vi "CreateMicron.vi"(8 "error in (no error)":errorcluster, 10 "New Microservice Name":string, 11 "Root Directory":path) -> (0 "error out":errorcluster, 3 "Project Path Out":path)   [LabVIEW 2019]
uses:
  <vilib>/SLL Toolkit/SLL Scripting/_Typedefs/Rename Item Cluster.ctl
  <vilib>/SLL Toolkit/SLL Scripting/SLL Scripting.lvlib
  <vilib>/SLL Toolkit/SLL Debug/SLL Debug.lvlib
panel:
  out "Micron Template Project Path":path
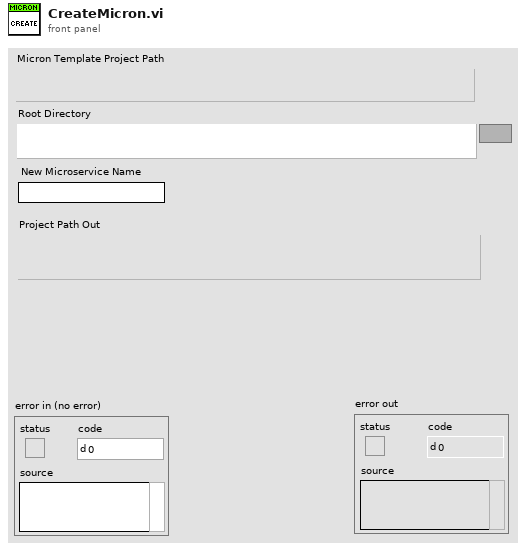
[diagram p1: front panel]
types:
  T1 = cluster{"Microservice Name":string, "Root Directory":path}
  T2 = typedef "SLL Scripting.lvlib/Rename Item Cluster.ctl" = cluster{"Existing":string, "Rename As":string}
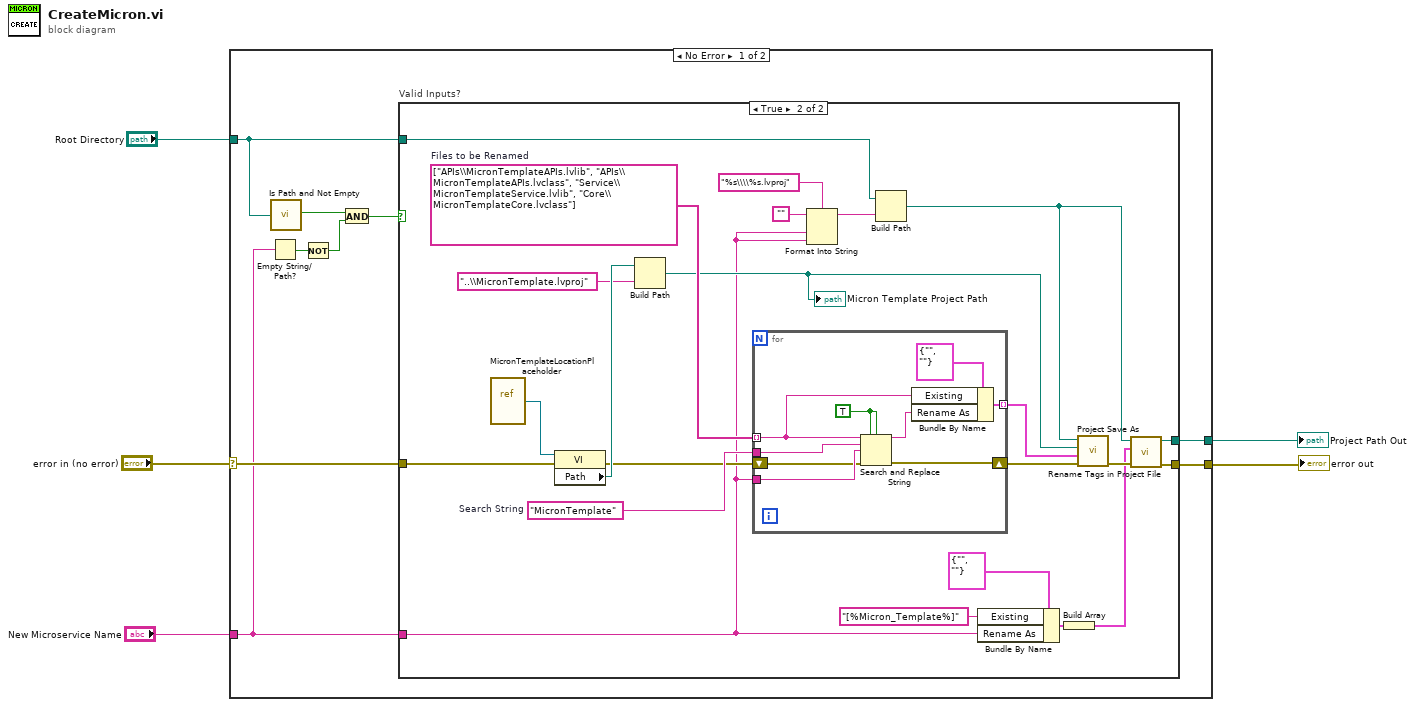
[diagram p0: block diagram]
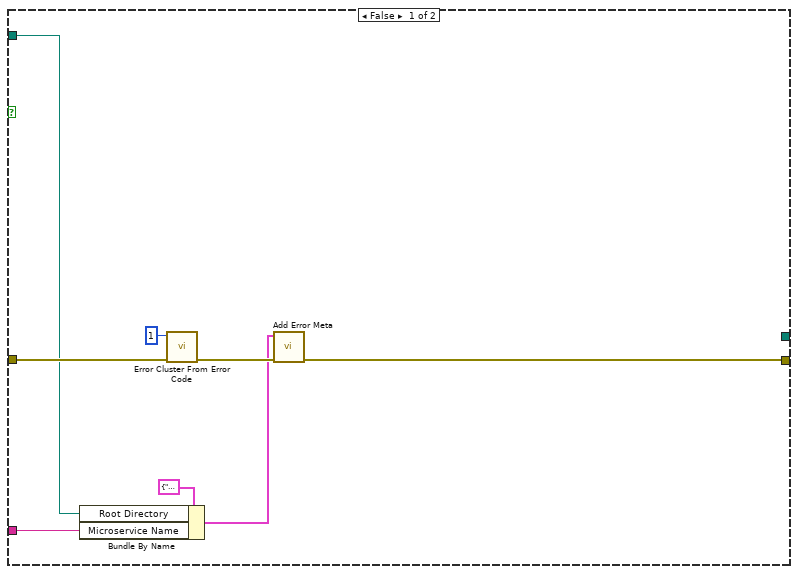
[diagram p2: hidden frame]
diagram:
  n1 = case shown="No Error" "error in (no error)" {
    selector: "error in (no error)" -> [w13 w55]
    tunnel: "Root Directory" -> [w11 _]
    tunnel: [w14 w55] -> w4
    tunnel: "New Microservice Name" -> [w10 _]
    tunnel: [w12 _] -> w1
    frame No Error {
      n2 = Empty String/Path?(string/path=w10) -> (empty?=w9:bool)
      n3 = call <vilib>:"Is Path and Not Empty.vi"("path"=w11) -> ("Is Path and Not Empty?"=w8:bool)  [unwired: 4 in]
      n4 = Not(x=w9) -> (.not. x?=w7:bool)
      n5 = And(x=w8, y=w7) -> (x .and. y?=w6:bool)
      n6 = case "Valid Inputs?" shown="True" w6 {
        tunnel: [w19 w37] -> w14
        tunnel: w13 -> [w22 w26]
        tunnel: [_ w25] -> w12
        tunnel: w11 -> [w17 w24]
        tunnel: w10 -> [w16 w23]
        frame False {
          n7 = Bundle By Name(cluster=T1 {"Microservice Name"="", "Root Directory"=path ""}, "Root Directory"=w17, "Microservice Name"=w16) -> (w15:T1)
          n8 = call <vilib>:"Error Cluster From Error Code.vi"("error in (no error)"=w22, "error code (0)"=1) -> ("error out"=w21:errorcluster)  [unwired: 7 in]
          n9 = call <vilib>:"Add Error Meta.vi"("error in (no error)"=w21, "Data"=w15) -> ("error out"=w19:errorcluster)  [unwired: 9 in]
        }
        frame True {
          w44 = "MicronTemplate"  # Search String
          w45 = string[] ["APIs\\MicronTemplateAPIs.lvlib", "APIs\\MicronTemplateAPIs.lvclass", "Service\\MicronTemplateService.lvlib", "Core\\MicronTemplateCore.lvclass"]  # Files to be Renamed
          n10 = vi-ref "MicronTemplateLocationPlaceholder.vi"() -> (w31:refnum<vi>)
          n11 = property class="VI"(reference=w31, error in=w26) -> (error out=w27:errorcluster, "Path"=w30:path)  [unwired: 1 out]
          n12 = Build Path(base path=w30, name or relative path="..\\MicronTemplate.lvproj") -> (appended path=w28:path)
          "Micron Template Project Path" <- w28
          n13 = for {
            tunnel: w45 -> [w50] mode=indexing
            tunnel: w44 -> [w54]
            tunnel: w23 -> [w53]
            tunnel: [w48] -> w43 mode=indexing
            shift-right: [w47] -> w42
            shift-left: w27 -> [w46]
            w52 = TRUE ("replace all? (F)")
            n14 = Search and Replace String(replace all?=w52, case sensitive?=w52, input string=w50, search string=w54, replace string=w53, error in=w46) -> (result string=w49:string, error out=w47:errorcluster)  [unwired: 2 in, 2 out]
            n15 = Bundle By Name(cluster=T2 {"Existing"="", "Rename As"=""} ("Rename Item"), "Existing"=w50, "Rename As"=w49) -> (w48:T2)
          }
          n16 = Format Into String(format string="%s\\\\%s.lvproj", initial string="", w23, w23) -> (resulting string=w41:string)  [unwired: 1 in, 1 out]
          n17 = Build Path(base path=w24, name or relative path=w41) -> (appended path=w36:path)
          n18 = Bundle By Name(cluster=T2 {"Existing"="", "Rename As"=""} ("Rename Item"), "Existing"="[%Micron_Template%]", "Rename As"=w23) -> (w33:T2)
          n19 = Build Array(w33) -> (w32:T2[])
          n20 = call <vilib>:"Project Save As.vi"("error in (no error)"=w42, "Rename Paths[]"=w43, "Existing Project Path"=w28, "New Project Path"=w36) -> ("error out"=w38:errorcluster)  [unwired: 7 in]
          n21 = call <vilib>:"Rename Tags in Project File.vi"("error in (no error)"=w38, "Rename Tags[]"=w32, "Project Path"=w36) -> ("error out"=w37:errorcluster, "Project Path Out"=w25:path)  [unwired: 7 in]
        }
      }
    }
    frame Error {
    }
  }
  "error out" <- w4
  "Project Path Out" <- w1
